vi "get rx antenna.vi"(8 "error in":errorcluster, 11 "MultiUsrp in":refnum<class "MultiUsrp.lvclass">) -> (0 "error out":errorcluster, 2 "ant_out out":string, 3 "MultiUsrp out":refnum<class "MultiUsrp.lvclass">)   [LabVIEW 2023, in "uhd.lvlib" / "MultiUsrp.lvclass"]
uses:
  <userlib>/uhd/MultiUsrp/MultiUsrp.lvclass
  <userlib>/uhd/MultiUsrp/MultiUsrp.lvclass/MultiUsrp.ctl
  <userlib>/uhd/uhd.lvlib
panel:
  in  "chan":u64
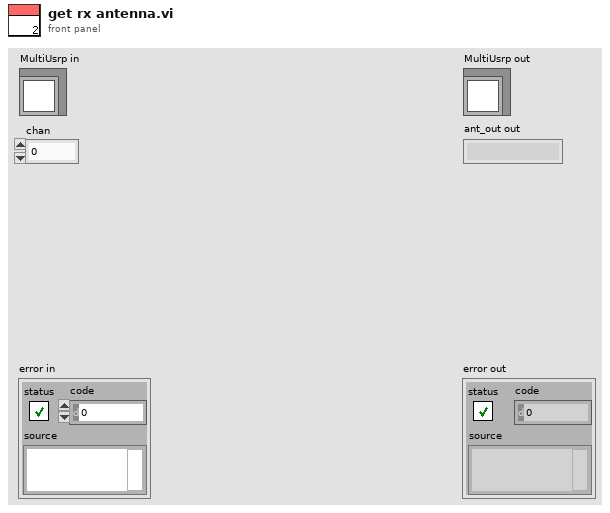
[diagram p1: front panel]
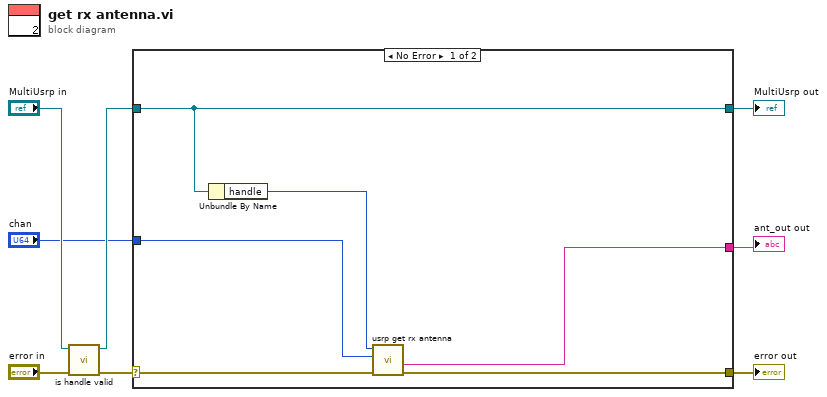
[diagram p0: block diagram]
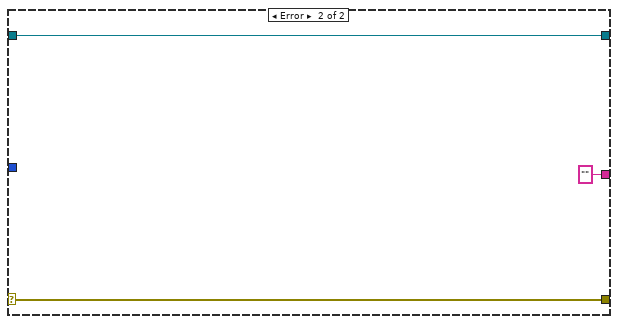
[diagram p2: hidden frame]
diagram:
  n1 = call <userlib>:"is handle valid.vi"("error in (no error)"="error in", "MultiUsrp in"="MultiUsrp in") -> ("error out"=w5:errorcluster, "MultiUsrp out"=w3:refnum<class "MultiUsrp.lvclass">)  [unwired: 8 in]
  n2 = case shown="No Error" w5 {
    selector: w5 -> [w14 w17]
    tunnel: [w13 w17] -> w8
    tunnel: [w11 w16] -> w7
    tunnel: w3 -> [w11 w16]
    tunnel: "chan" -> [w12 _]
    tunnel: [w9 "" ("ant_out out")] -> w1
    frame No Error {
      n3 = Unbundle By Name(w11) -> ("handle"=w10:u64)
      n4 = call <userlib>:"usrp get rx antenna.vi"("error in (no error)"=w14, "chan"=w12, "h"=w10) -> ("error out"=w13:errorcluster, "ant_out out"=w9:string)  [unwired: 6 in, 1 out]
    }
    frame Error {
    }
  }
  "error out" <- w8
  "MultiUsrp out" <- w7
  "ant_out out" <- w1
